vi "Insert.vi"(6 "can be indented? (T)":bool=TRUE, 9 "insert":string, 10 "sections":string[](array[string]), 11 "info data":string) -> (3 "info data out":string)   [LabVIEW 2019, in "infolib.lvlib"]
doc: "Inserts key or table into sections structure and appends to the string. If sections structure already exist, inserts at the end of the required section."
uses:
  infolib.lvlib
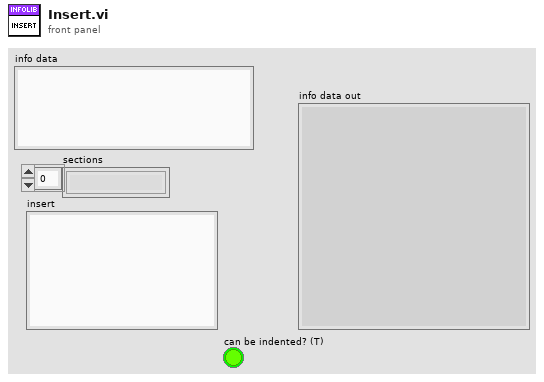
[diagram p1: front panel]
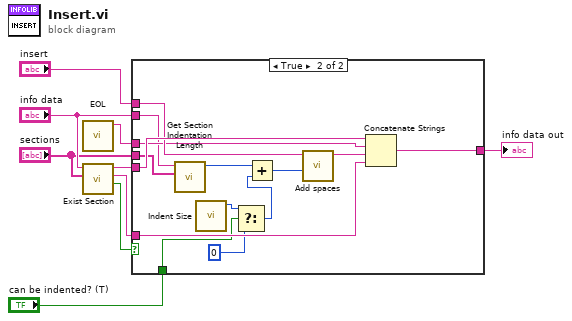
[diagram p0: block diagram]
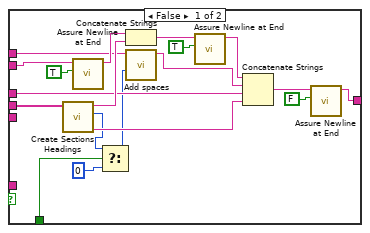
[diagram p2: hidden frame]
diagram:
  n1 = call "EOL.vi"() -> ("eol"=w2:string)  [unwired: 11 in]
  n2 = call "Exist Section.vi"("sections"="sections", "info data"="info data") -> ("exist"=w4:bool, "after end of section"=w7:string, "before end of section"=w6:string)  [unwired: 7 in]
  n3 = case shown="True" w4 {
    tunnel: "sections" -> [w28 w36]
    tunnel: w6 -> [_ w42]
    tunnel: w7 -> [_ w41]
    tunnel: "insert" -> [w15 w38]
    tunnel: [w17 w40] -> w8
    tunnel: "info data" -> [w27 w35]
    tunnel: w2 -> [w19 w37]
    tunnel: "can be indented? (T)" -> [w13 w29]
    frame False {
      n4 = call "Create Sections Headings.vi"("sections"=w28) -> ("sections end"=w25:string, "spaces number"=w12:i32, "sections start"=w23:string)  [unwired: 8 in]
      n5 = call "Assure Newline at End.vi"("Set End Of Line (F)"=TRUE ("newline"), "string"=w27) -> ("string out"=w24:string)  [unwired: 9 in]
      n6 = Select(t=w12, s=w13, f=0) -> (s? t:f=w11:i32)
      n7 = Concatenate Strings(w24, w23) -> (w20:string)
      n8 = call "Add spaces.vi"("spaces no"=w11, "input string"=w15) -> ("result string"=w14:string)  [unwired: 9 in]
      n9 = call "Assure Newline at End.vi"("Set End Of Line (F)"=TRUE ("newline"), "string"=w20) -> ("string out"=w22:string)  [unwired: 9 in]
      n10 = Concatenate Strings(w22, w14, w19, w25) -> (w18:string)
      n11 = call "Assure Newline at End.vi"("Set End Of Line (F)"=FALSE ("End Of Line (F)"), "string"=w18) -> ("string out"=w17:string)  [unwired: 9 in]
    }
    frame True {
      n12 = call "Get Section Indentation Length.vi"("sections"=w36, "info data"=w35) -> ("Indentation length"=w34:i32)  [unwired: 9 in]
      n13 = call "Indent Size.vi"() -> ("indent size"=w32:i32)  [unwired: 10 in, 1 out]
      n14 = Select(t=w32, s=w29, f=0) -> (s? t:f=w31:i32)
      n15 = Add(x=w34, y=w31) -> (x+y=w33:i32)
      n16 = call "Add spaces.vi"("spaces no"=w33, "input string"=w38) -> ("result string"=w39:string)  [unwired: 9 in]
      n17 = Concatenate Strings(w42, w37, w39, w41) -> (w40:string)
    }
  }
  "info data out" <- w8
